vi "NI 9260 Generate Signal (FPGA).vi"() -> ()   [LabVIEW 2021]
uses:
  <vilib>/LabVIEW Targets/FPGA/cRIO/shared/nicrio_ModuleControls/nicrio_cRIO-9260_DataRatesRing2.ctl
  <vilib>/rvi/Emulation/niFpgaGetClockAttributes.vi
  <vilib>/rvi/Emulation/niFpgaSctlEmulationGetInTimedLoop.vi
  <vilib>/rvi/Emulation/niFpgaEmulationReportErrorSimple.vi
  <vilib>/rvi/eio/common/nirviEmuTemplatePropertySet_errors.vi
  <vilib>/rvi/eio/common/nirviEmuTemplateMethod_errors.vi
  <vilib>/rvi/interface/RandomDataEmulation/niFpgaRandomDataHandleErrors.vi
  <vilib>/rvi/Emulation/niFpgaCriticalErrorInLSC.vi
  <vilib>/eio/EIOPropertyNode/EIOPropertyNode.xnode
  <vilib>/eio/EIONode/EIONode.xnode
  <vilib>/rvi/DataTransferAndStorage/Container/XNode/niFpgaContainer.xnode
  <vilib>/rvi/interface/RandomDataEmulation/nirviRandomDataFpgaReadWriteTemplate.vi
  <vilib>/eio/EIOMethodNode/EIOMethodNode.xnode
  <vilib>/rvi/eio/common/nirviEmuTemplatePropertyGet_errors.vi
  <vilib>/rvi/eio/common/nirviEmuTemplatePropertyGet_noerrors.vi
  <vilib>/rvi/eio/common/nirviEmuTemplatePropertySet_noerrors.vi
panel:
  in  "stop":bool
  out "FIFO Time Out":bool
  in  "Data Rate":T1=1 items=["51.200 kS/s (NI 9260)"=1, "25.600 kS/s (NI 9260)"=2, "17.067 kS/s (NI 9260)"=3, "12.800 kS/s (NI 9260)"=4, "10.240 kS/s (NI 9260)"=5, "8.533 kS/s (NI 9260)"=6, "7.314 kS/s (NI 9260)"=7, "6.400 kS/s (NI 9260)"=8, "5.689 kS/s (NI 9260)"=9, "5.120 kS/s (NI 9260)"=10, "4.654 kS/s (NI 9260)"=11, "4.267 kS/s (NI 9260)"=12, "3.938 kS/s (NI 9260)"=13, "3.657 kS/s (NI 9260)"=14, "3.413 kS/s (NI 9260)"=15, "3.200 kS/s (NI 9260)"=16, "3.012 kS/s (NI 9260)"=17, "2.845 kS/s (NI 9260)"=18, "2.695 kS/s (NI 9260)"=19, "2.560 kS/s (NI 9260)"=20, "2.438 kS/s (NI 9260)"=21, "2.328 kS/s (NI 9260)"=22, "2.226 kS/s (NI 9260)"=23, "2.133 kS/s (NI 9260)"=24, "2.048 kS/s (NI 9260)"=25, "1.969 kS/s (NI 9260)"=26, "1.896 kS/s (NI 9260)"=27, "1.829 kS/s (NI 9260)"=28, "1.765 kS/s (NI 9260)"=29, "1.707 kS/s (NI 9260)"=30, "1.652 kS/s (NI 9260)"=31]
  out "Overvoltage":bool[](array[boolean])
  out "Underflow":bool[](array[boolean])
  out "FPGA Error out":errorcluster
  # "Overview: Demonstrates how to generate a sine wave from the NI 9260\nRequirements: LabVIEW Full Development System, LV FPGA, and NI RIO\nInstructions: \n1. Run NI 9260 Getting Started (Host).vi"
  # "Output Parameters"
  # "Input Parameters"
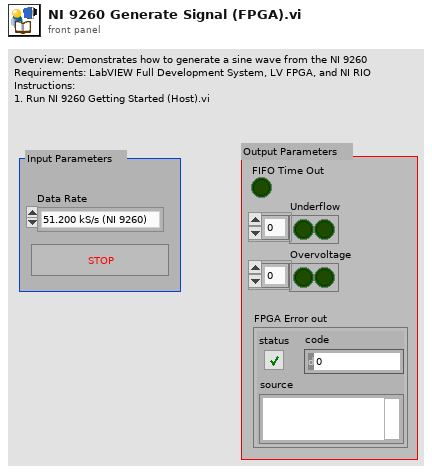
[diagram p1: front panel]
types:
  T1 = typedef "nicrio_cRIO-9260_DataRatesRing2.ctl" = u8
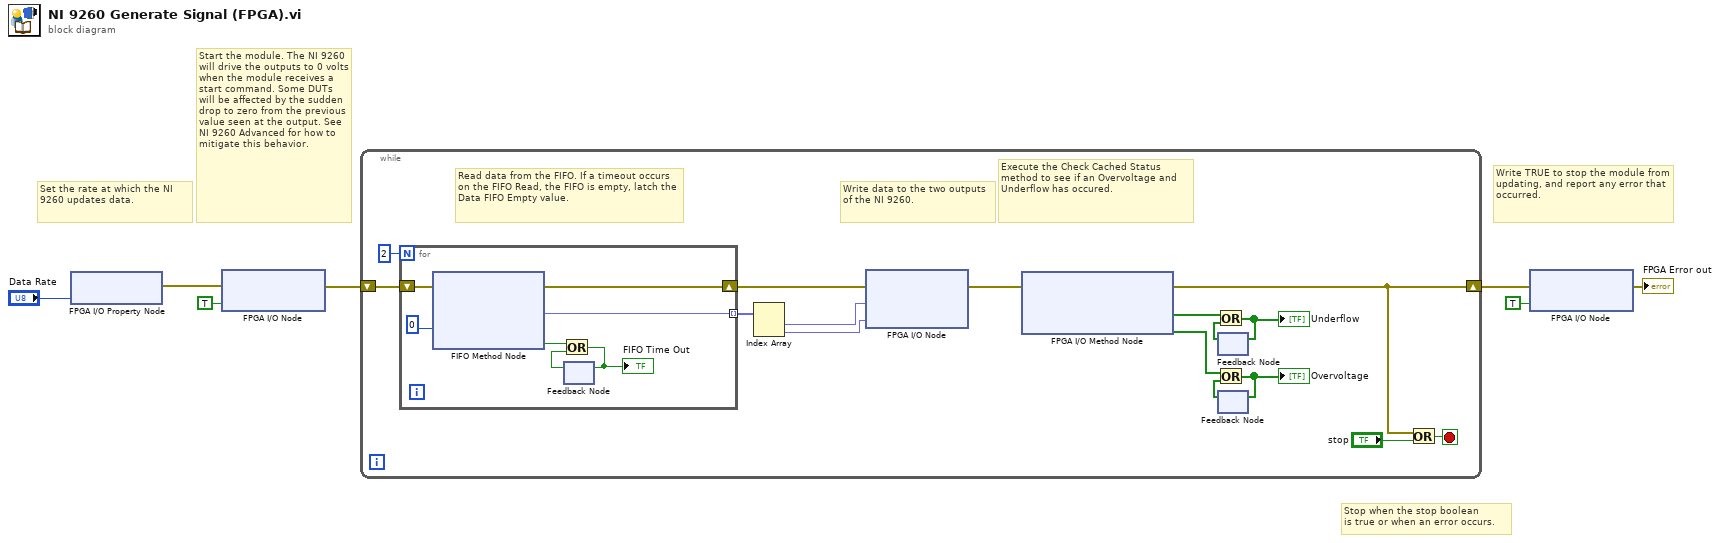
[diagram p0: block diagram]
diagram:
  # "Stop when the stop boolean\nis true or when an error occurs."
  # "Write TRUE to stop the module from updating, and report any error that occurred."
  # "Start the module. The NI 9260 will drive the outputs to 0 volts when the module receives a start command. Some DUTs will be affected by the sudden drop to zero from the previous value seen at the output. See NI 9260 Advanced for how to mitigate this behavior."
  # "Set the rate at which the NI 9260 updates data."
  n1 = xnode "FPGA I/O Property Node"("Data Rate"="Data Rate") -> ("error out"=w7:errorcluster)  [unwired: 2 in, 1 out]
  n2 = xnode "FPGA I/O Node"("error in"=w7, "Mod4/Start"=TRUE ("Mod1/Start")) -> ("error out"=w6:errorcluster)  [unwired: 1 in, 1 out]
  n3 = while {
    shift-right: [w19] -> w3
    shift-left: w6 -> [w22]
    stop <- w20 stop-if-true
    # "Read data from the FIFO. If a timeout occurs on the FIFO Read, the FIFO is empty, latch the Data FIFO Empty value."
    # "Execute the Check Cached Status method to see if an Overvoltage and Underflow has occured."
    # "Write data to the two outputs of the NI 9260."
    n4 = for {
      N: 2 -> [_]
      tunnel: [w24] -> w16 mode=indexing
      shift-right: [w25] -> w21
      shift-left: w22 -> [w26]
      n5 = xnode ("FIFO Method Node")("Timeout"=0, "error in (no error)"=w26) -> ("Element"=w24:fxp<+/-,24,4>, "Timed Out?"=w29:bool, "error out"=w25:errorcluster)  [unwired: 1 in, 1 out]
      n6 = feedback #1() -> (w27:bool)  [unwired: 1 in]
      n7 = Or(x=w29, y=w27) -> (x .or. y?=w28:bool)
      "FIFO Time Out" <- w28
      n8 = feedback-in #1(w28) -> ()
    }
    n9 = Index Array(array=w16) -> (element #1=w15:fxp<+/-,24,4>, element #2=w14:fxp<+/-,24,4>)  [unwired: 2 in]
    n10 = xnode "FPGA I/O Node"("error in"=w21, "Mod4/AO0"=w15, "Mod4/AO1"=w14) -> ("error out"=w23:errorcluster)  [unwired: 2 in, 2 out]
    n11 = xnode "FPGA I/O Method Node"("error in"=w23) -> ("error out"=w19:errorcluster, "Underflow"=w12:bool[], "Overvoltage"=w11:bool[])  [unwired: 1 in, 1 out]
    n12 = feedback #2() -> (w13:bool[])  [unwired: 1 in]
    n13 = Or(x=w12, y=w13) -> (x .or. y?=w9:bool[])
    "Underflow" <- w9
    n14 = feedback-in #2(w9) -> ()
    n15 = feedback #3() -> (w10:bool[])  [unwired: 1 in]
    n16 = Or(x=w11, y=w10) -> (x .or. y?=w8:bool[])
    "Overvoltage" <- w8
    n17 = feedback-in #3(w8) -> ()
    n18 = Or(x=w19, y="stop") -> (x .or. y?=w20:bool)
  }
  n19 = xnode "FPGA I/O Node"("error in"=w3, "Mod4/Stop"=TRUE ("Mod1/Stop")) -> ("error out"=→"FPGA Error out":errorcluster)  [unwired: 1 in, 1 out]
